vi "Close.vi"(8 "error in (no error)":errorcluster, 11 "Progress Bar":refnum<data-value>) -> (0 "error out":errorcluster)   [LabVIEW 2020, in "Progress Bar.lvclass"]
doc: "Call this VI after the loop to dispose of all references\n\nCopyright: MGI\nAuthored by: Derek Trepanier"
uses:
  <userlib>/_MGI/User Interface/Progress Bar/Progress Bar.lvclass
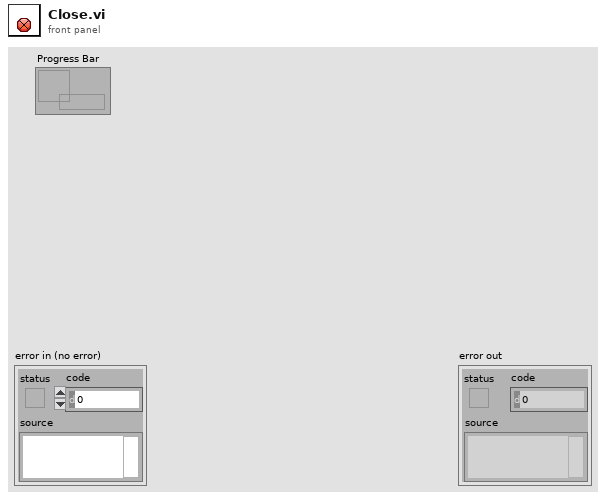
[diagram p1: front panel]
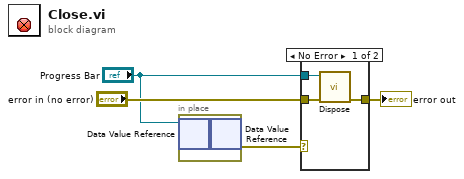
[diagram p0: block diagram]
diagram:
  n1 = in-place {
    n2 = in-place-dvr #1("Progress Bar") -> (w5:refnum<class "Progress Bar.lvclass">)  [unwired: 1 out]
    n3 = in-place-dvr #1(w5) -> (w1:errorcluster)  [unwired: 1 out]
  }
  n4 = case shown="No Error" w1 {
    tunnel: "Progress Bar" -> [w8 _]
    tunnel: "error in (no error)" -> [w7 w9]
    tunnel: [w6 w9] -> w3
    frame No Error {
      n5 = call <userlib>:"Dispose.vi"("error in (no error)"=w7, "Data Value Reference in"=w8) -> ("error out"=w6:errorcluster)  [unwired: 9 in]
    }
    frame Error {
    }
  }
  "error out" <- w3
